vi "LVClasse_Surface Set Data.vi"(0 "SurfaceFloat in":refnum<class "Surface.lvclass">, 5 "data":sgl[][](array[numeric]), 11 "error in (no error)":errorcluster) -> (4 "SurfaceFloat out":refnum<class "Surface.lvclass">, 15 "error out":errorcluster)   [LabVIEW 2020, in "Surface.lvclass"]
doc: "Get write access Surface buffer.\n\n--------------------------------------------------------------------------------\n\n<B>SurfaceIn </B> : Surface object.\n<B>SurfaceOut </B> : Surface object.\n<B>data </B> : Surface buffer to set.\n<B>ErrorIn </B> : Error\n<B>ErrorOut </B> : Error\n\n--------------------------------------------------------------------------------"
uses:
  Surface.lvclass
  Surface.lvclass/Surface.ctl
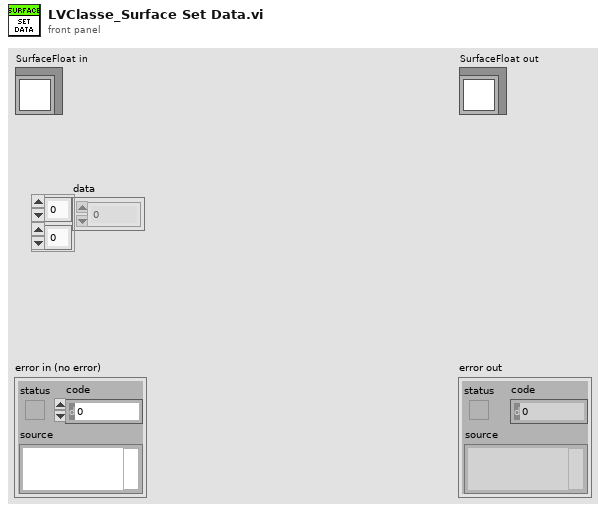
[diagram p1: front panel]
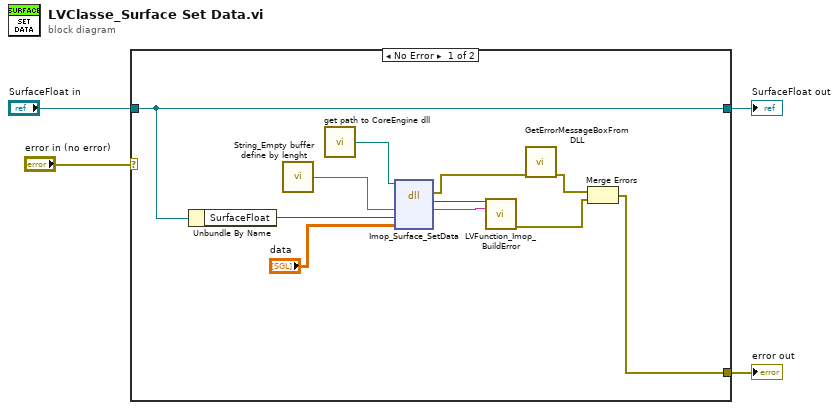
[diagram p0: block diagram]
diagram:
  n1 = case shown="No Error" "error in (no error)" {
    selector: "error in (no error)" -> [_ w17]
    tunnel: [w5 w17] -> w4
    tunnel: [w10 w16] -> w3
    tunnel: "SurfaceFloat in" -> [w10 w16]
    frame No Error {
      n2 = Unbundle By Name(w10) -> ("SurfaceFloat"=w9:i32)
      n3 = call "String_Empty buffer define by lenght.vi"() -> ("Empty buffer"=w13:string)  [unwired: 1 in]
      n4 = call "get path to CoreEngine dll.vi"() -> ("path to c_interface_vc100.dll"=w12:path)  [unwired: 12 in, 3 out]
      n5 = dll-call lib="D:/2_trunk/Soft_haso/ImOpCoreEngine4_LV2011/DLLs/ImopEngine4_vc100.dll" fn="Imop_Surface_SetData"(path in=w12, "message"=w13, "surface"=w9, "data"="data") -> (error out=w11:errorcluster, "return type"=w15:i32, "message"=w14:string)  [unwired: 4 in, 1 out]
      n6 = call "LVFunction_Imop_BuildError.vi"("code"=w15, "String to Prepend to source (\"\")"=w14) -> ("error out"=w6:errorcluster)  [unwired: 13 in]
      n7 = call "GetErrorMessageBoxFromDLL.vi"("error IN"=w11) -> ("error OUT"=w7:errorcluster)  [unwired: 10 in]
      n8 = Merge Errors(w7, w6) -> (w5:errorcluster)
    }
    frame Error {
    }
  }
  "error out" <- w4
  "SurfaceFloat out" <- w3
